vi "Get Project Members.vi"(6 "Authorization":T2[](array[typedef]), 8 "error in (no error)":errorcluster, 11 "Project GID":string) -> (0 "error out":errorcluster, 3 "data":T1(array[cluster]))   [LabVIEW 2016]
uses:
  <vilib>/addons/_JKI.lib/REST Client/classes/REST Client/HTTP Header.ctl
  <vilib>/addons/_JKI.lib/REST Client/classes/REST Client/REST Client.lvclass
  <vilib>/addons/_JKI.lib/Serialization/JSON/JKI JSON Serialization.lvlib
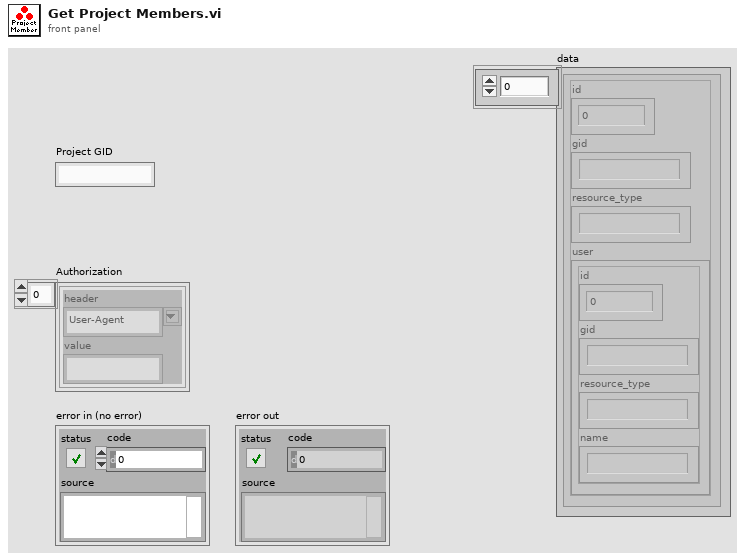
[diagram p1: front panel]
types:
  T1 = cluster{"id":i32, "gid":string, "resource_type":string, "user":cluster{"id":i32, "gid":string, "resource_type":string, "name":string}}[]
  T2 = typedef "REST Client.lvlib/REST Client.lvclass/HTTP Header.ctl" = cluster{"header":string, "value":string}
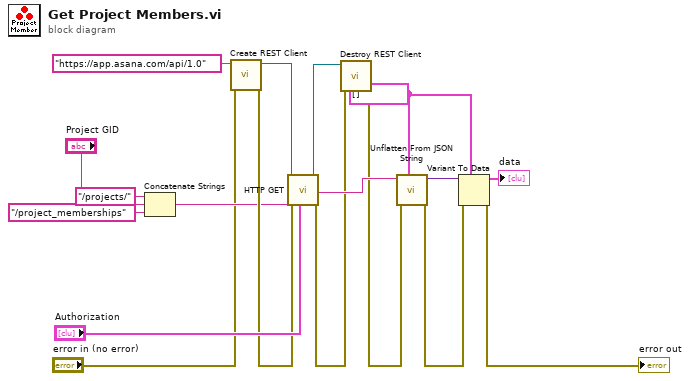
[diagram p0: block diagram]
diagram:
  w2 = T1 []
  n1 = Concatenate Strings("/projects/" ("string"), "Project GID", "/project_memberships" ("string")) -> (w12:string)
  n2 = call <vilib>:"Create REST Client.vi"("error in (no error)"="error in (no error)", "Base URL"="https://app.asana.com/api/1.0") -> ("error out"=w15:errorcluster, "REST Client out"=w18:refnum<class "REST Client.lvclass">)  [unwired: 8 in]
  n3 = call-dynamic "HTTP GET.vi"("request specific headers"="Authorization", "error in (no error)"=w15, "Path"=w12, "REST Client in"=w18) -> ("error out"=w7:errorcluster, "Response body"=w9:string, "REST Client out"=w17:refnum<class "REST Client.lvclass">)  [unwired: 2 in, 3 out]
  n4 = call-dynamic "Destroy REST Client.vi"("error in (no error)"=w7, "REST Client in"=w17) -> ("error out"=w6:errorcluster)  [unwired: 9 in]
  n5 = call <vilib>:"Unflatten From JSON String.vi"("Type and Defaults"=w2, "error in (no error)"=w6, "JSON String"=w9) -> ("error out"=w5:errorcluster, "Variant"=w8:variant)  [unwired: 7 in]
  n6 = Variant To Data(error in=w5, type=w2, Variant=w8) -> (data=→"data":T1, error out=→"error out":errorcluster)
